vi "VisualInspection.vi"(8 "error in (no error)":errorcluster, 11 "TableRef":refnum<vi>) -> (0 "error out":errorcluster)   [LabVIEW 2017]
panel:
  in  "Cancel Button":bool
  in  "OK Button":bool
  in  "7.5.1.1":bool
  in  "7.3":bool
  in  "7.2.3":bool
  in  "7.2.4":bool
  in  "7.2.5":bool
  in  "6.2.2.1":bool
  in  "6.2.2.2":bool
  in  "6.2.2.3":bool
  in  "6.2.2.4":bool
  in  "7.1":bool
  in  "6.2.1.1":bool
  in  "7.2.2":bool
  in  "6.1.2":bool
  in  "7.2.1.1":bool
  in  "7.2.1":bool
  in  "6.1.1":bool
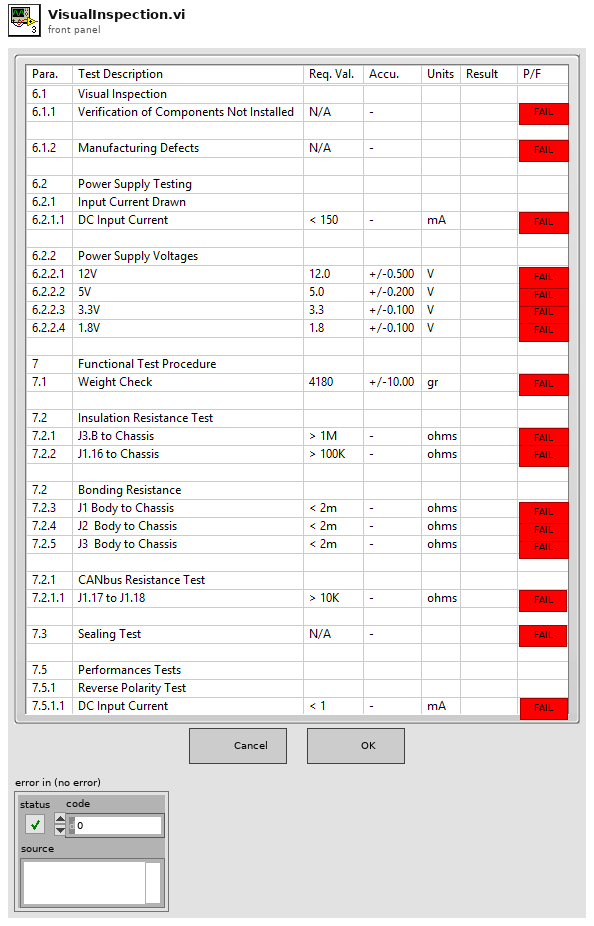
[diagram p1: front panel]
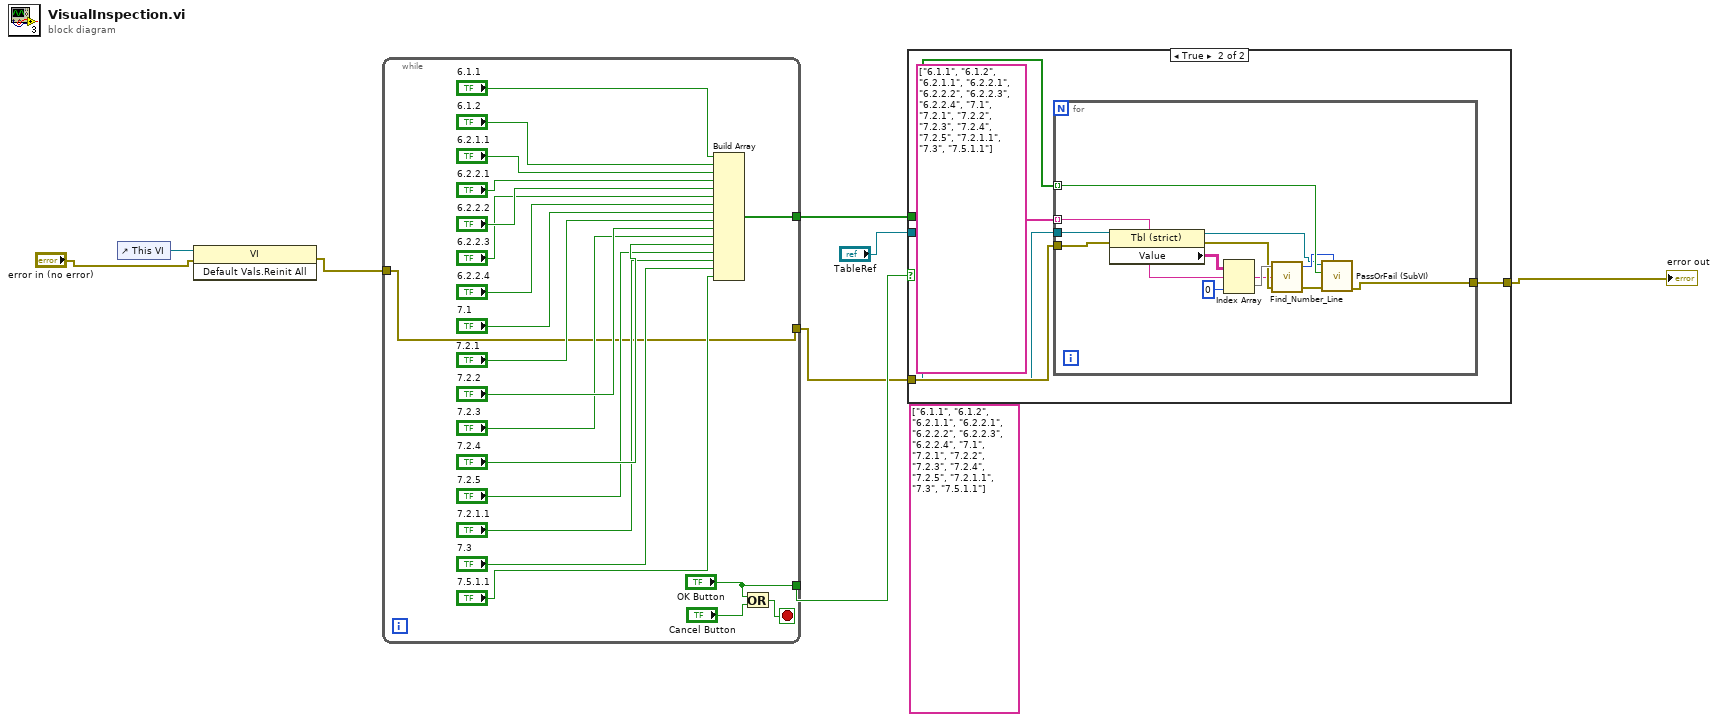
[diagram p0: block diagram]
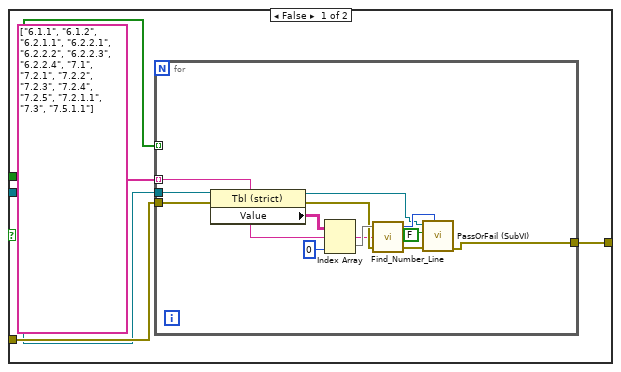
[diagram p2: hidden frame]
diagram:
  (unwired) string[] ["6.1.1", "6.1.2", "6.2.1.1", "6.2.2.1", "6.2.2.2", "6.2.2.3", "6.2.2.4", "7.1", "7.2.1", "7.2.2", "7.2.3", "7.2.4", "7.2.5", "7.2.1.1", "7.3", "7.5.1.1"]
  n1 = control-ref of="This VI"() -> (w3:refnum<vi>)
  n2 = invoke class="VI" method="Default Vals.Reinit All"(reference=w3, error in="error in (no error)") -> (error out=w8:errorcluster)  [unwired: 1 in, 2 out]
  n3 = while {
    tunnel: w8 -> [w9]
    tunnel: [w11] -> w7
    tunnel: ["OK Button"] -> w6
    tunnel: [w9] -> w5
    stop <- w28 stop-if-true
    n4 = Build Array("6.1.1", "6.1.2", "6.2.1.1", "6.2.2.1", "6.2.2.2", "6.2.2.3", "6.2.2.4", "7.1", "7.2.1", "7.2.2", "7.2.3", "7.2.4", "7.2.5", "7.2.1.1", "7.3", "7.5.1.1") -> (w11:bool[])
    n5 = Or(x="OK Button", y="Cancel Button") -> (x .or. y?=w28:bool)
  }
  n6 = case shown="True" w6 {
    tunnel: w7 -> [w33 w50]
    tunnel: w5 -> [w32 w49]
    tunnel: [w31 w48] -> w1
    tunnel: "TableRef" -> [w30 w47]
    frame False {
      n7 = for {
        tunnel: string[] ["6.1.1", "6.1.2", "6.2.1.1", "6.2.2.1", "6.2.2.2", "6.2.2.3", "6.2.2.4", "7.1", "7.2.1", "7.2.2", "7.2.3", "7.2.4", "7.2.5", "7.2.1.1", "7.3", "7.5.1.1"] -> [w42] mode=indexing
        tunnel: w33 -> [_] mode=indexing
        tunnel: w32 -> [w38]
        tunnel: [w37] -> w31
        tunnel: w30 -> [w36]
        n8 = property class="Tbl (strict)"(reference=w36, error in=w38) -> (reference out=w39:refnum<vi>, error out=w43:errorcluster, "Value"=w46:string[][])
        n9 = Index Array(array=w46, index (col)=0 ("disabled index (col)")) -> (element=w44:string[])  [unwired: 1 in]
        n10 = call "Find_Number_Line.vi"("error in"=w43, "Test Paragraph"=w42, "Row Headers[]"=w44) -> ("error out"=w41:errorcluster, "Line number"=w40:i32)  [unwired: 1 out]
        n11 = call "PassOrFail (SubVI).vi"("index (row)"=w40, "error in (no error)"=w41, "Pass?Fail"=FALSE ("Boolean"), "Table in"=w39) -> ("error out"=w37:errorcluster)  [unwired: 7 in]
      }
    }
    frame True {
      n12 = for {
        tunnel: string[] ["6.1.1", "6.1.2", "6.2.1.1", "6.2.2.1", "6.2.2.2", "6.2.2.3", "6.2.2.4", "7.1", "7.2.1", "7.2.2", "7.2.3", "7.2.4", "7.2.5", "7.2.1.1", "7.3", "7.5.1.1"] -> [w59] mode=indexing
        tunnel: w50 -> [w57] mode=indexing
        tunnel: w49 -> [w54]
        tunnel: [w53] -> w48
        tunnel: w47 -> [w52]
        n13 = property class="Tbl (strict)"(reference=w52, error in=w54) -> (reference out=w55:refnum<vi>, error out=w60:errorcluster, "Value"=w63:string[][])
        n14 = Index Array(array=w63, index (col)=0 ("disabled index (col)")) -> (element=w61:string[])  [unwired: 1 in]
        n15 = call "Find_Number_Line.vi"("error in"=w60, "Test Paragraph"=w59, "Row Headers[]"=w61) -> ("error out"=w58:errorcluster, "Line number"=w56:i32)  [unwired: 1 out]
        n16 = call "PassOrFail (SubVI).vi"("index (row)"=w56, "error in (no error)"=w58, "Pass?Fail"=w57, "Table in"=w55) -> ("error out"=w53:errorcluster)  [unwired: 7 in]
      }
    }
  }
  "error out" <- w1
